vi "SC TCP SoundCheck Run Seq and Wait for Completion.vi"(7 "TimeOut(s)":dbl=60.0, 8 "error in (no error)":errorcluster, 9 "Sequence to run (full path)":path, 10 "port (4444)":u16=4444, 11 "SoundCheck IP Address (localhost)":string="localhost") -> (0 "error out":errorcluster, 1 "Duration":dbl, 3 "Ran to completion":bool)   [LabVIEW 2018]
doc: "Allows the user to control the running of a SoundCheck sequence from their own LabVIEW application."
uses:
  Common/Utils/Errors/Error.Error Code List.ctl
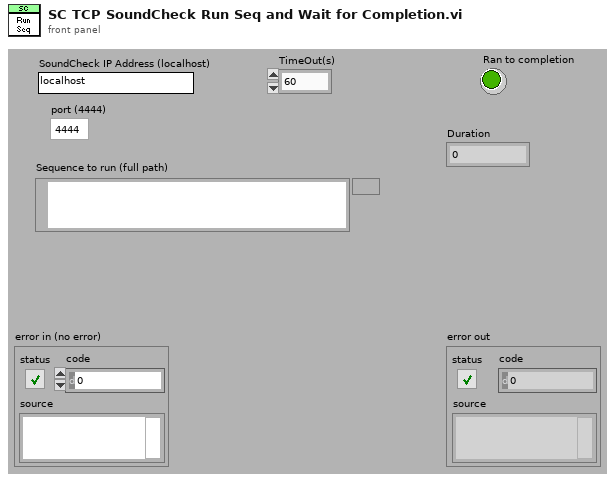
[diagram p1: front panel]
types:
  T1 = typedef "Error.Error Code List.ctl" = i32
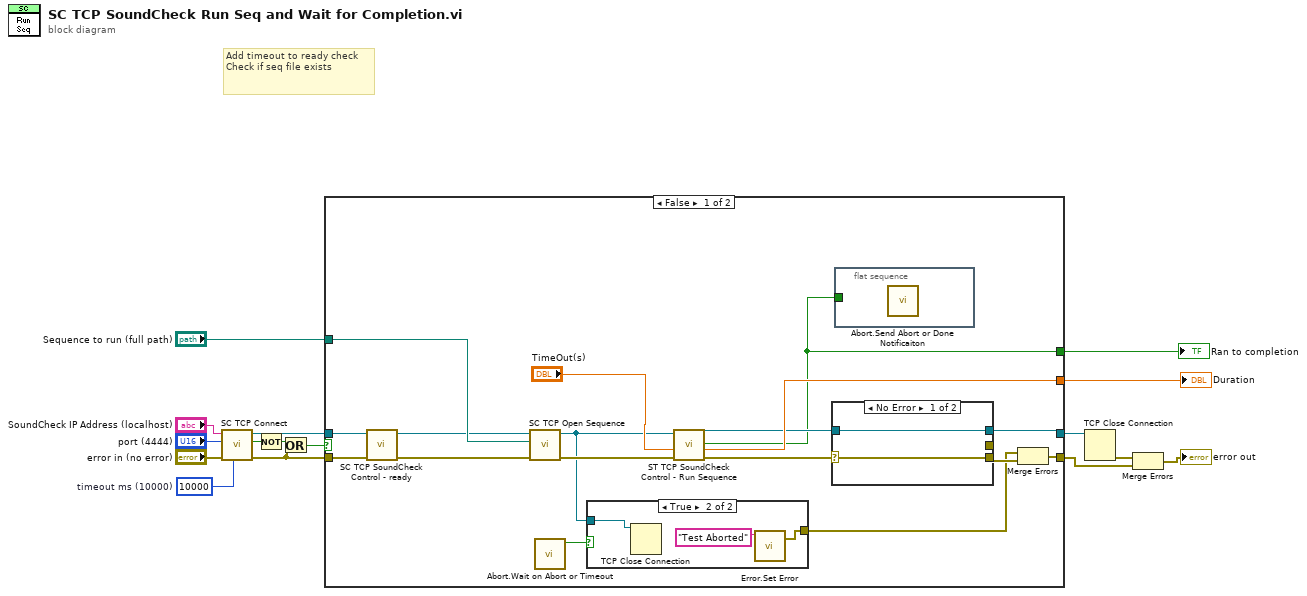
[diagram p0: block diagram]
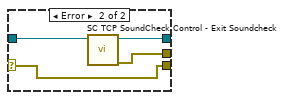
[diagram p3: hidden frame]
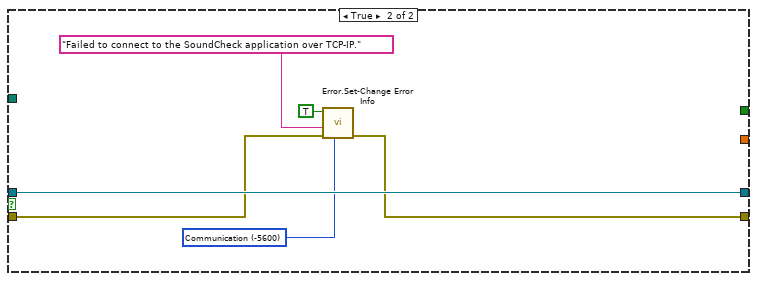
[diagram p4: hidden frame]
diagram:
  w1 = 10000  # timeout ms (10000)
  # "Add timeout to ready check\nCheck if seq file exists"
  n1 = call "SC TCP Connect.vi"("timeout ms (10000)"=w1, "error in (no error)"="error in (no error)", "port"="port (4444)", "Server IP Address"="SoundCheck IP Address (localhost)") -> ("error out"=w8:errorcluster, "Connected"=w9:bool, "TCP Network Connection out"=w12:refnum<k5>)  [unwired: 5 in]
  n2 = Not(x=w9) -> (.not. x?=w6:bool)
  n3 = Or(x=w6, y=w8) -> (x .or. y?=w7:bool)
  n4 = case shown="False" w7 {
    tunnel: [w19 w46] -> w2
    tunnel: [w20 _] -> w15
    tunnel: w12 -> [w32 w48]
    tunnel: [w26 _] -> w11
    tunnel: "Sequence to run (full path)" -> [w31 _]
    tunnel: w8 -> [w33 w47]
    tunnel: [w24 w48] -> w4
    frame False {
      n5 = call "SC TCP SoundCheck Control - ready.vi"("error in (no error)"=w33, "connection ID in"=w32) -> ("error out"=w29:errorcluster, "connection ID out"=w30:refnum<k5>)  [unwired: 7 in, 1 out]
      n6 = call "SC TCP Open Sequence.vi"("error in (no error)"=w29, "Sequence"=w31, "TCP Network Connection in"=w30) -> ("error out"=w28:errorcluster, "TCP Network Connection out"=w21:refnum<k5>)  [unwired: 7 in]
      n7 = call "Abort.Wait on Abort or Timeout.vi"() -> ("Abort"=w22:bool)  [unwired: 10 in, 1 out]
      n8 = case shown="True" w22 {
        tunnel: w21 -> [_ w36]
        tunnel: [_ w34] -> w17
        frame False {
        }
        frame True {
          n9 = TCP Close Connection(connection ID=w36) -> ()  [unwired: 2 in, 2 out]
          n10 = call "Error.Set Error.vi"("Desc"="Test Aborted") -> ("error out"=w34:errorcluster)  [unwired: 6 in]
        }
      }
      n11 = call "ST TCP SoundCheck Control - Run Sequence.vi"("error in (no error)"=w28, "TimeOut(s)"="TimeOut(s)", "TCP Cnct in"=w21) -> ("error out"=w23:errorcluster, "Duration"=w26:dbl, "Success?"=w20:bool, "TCP Cnct out"=w25:refnum<k5>)  [unwired: 5 in]
      n12 = case shown="No Error" w23 {
        selector: w23 -> [w37 w40]
        tunnel: w25 -> [w38 w42]
        tunnel: [w38 w41] -> w24
        tunnel: [w37 w40] -> w18
        tunnel: [_ w39] -> _
        frame No Error {
        }
        frame Error {
          n13 = call "SC TCP SoundCheck Control - Exit Soundcheck.vi"("TCP Network Connection in"=w42) -> ("error out"=w39:errorcluster, "TCP Network Connection out"=w41:refnum<k5>)  [unwired: 9 in]
        }
      }
      n14 = flat-sequence {
        tunnel: w20 -> [_]
        frame #0 {
          n15 = call "Abort.Send Abort or Done Notificaiton.vi"() -> ()  [unwired: 11 in, 1 out]
        }
      }
      n16 = Merge Errors(w17, w18) -> (w19:errorcluster)
    }
    frame True {
      w43 = T1 -5600 items=["No Error"=0, "Abort"=-2, "Misc"=-5000, "Fixture Error"=-5100, "File IO - General"=-5200, "FIle IO - Config Error"=-5201, "Instrument - General"=-5300, "Instrument - Serial Com"=-5301, "Instrument - Camera"=-5302, "Instrument - PS"=-5303, "Instrument - Oscilloscope"=-5304, "Instrument - Function Gen"=-5305, "Instrument - Load"=-5306, "Instrument - Meter"=-5307, "Instrument - Power Control"=-5308, "Instrument - Motion"=-5309, "Instrument - RF"=-5310, "System Exe"=-5400, "Image Processing"=-5500, "Communication"=-5600, "Script - Syntax Error"=-6000, "Script - Invalid Name or Param"=-6100, "Script - Timeout"=-6200, "Invalid Data"=-6300, "FW Update Error"=-6500] ("Std Code")
      n17 = call "Error.Set-Change Error Info.vi"("Std Code"=w43, "error in"=w47, "Description"="Failed to connect to the SoundCheck application over TCP-IP.", "Set Error"=TRUE) -> ("error out"=w46:errorcluster)  [unwired: 7 in]
    }
  }
  "Ran to completion" <- w15
  "Duration" <- w11
  n18 = TCP Close Connection(connection ID=w4) -> (error out=w5:errorcluster)  [unwired: 2 in, 1 out]
  n19 = Merge Errors(w5, w2) -> (→"error out":errorcluster)
